vi "write_text_file_temp.vi"(0 "counts":i32=124928 caption="photon count", 1 "name":string, 2 "base path":path) -> ()   [LabVIEW 2013]
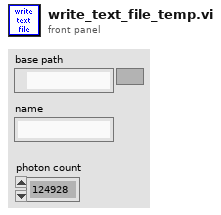
[diagram p1: front panel]
types:
  T1 = enum16{"open", "replace", "create", "open or create", "replace or create", "replace or create with confirmation"}
  T2 = cluster{"Xpixels":i32, "Vx-min ref":dbl, "Vx-max ref":dbl, "P":dbl, "Ypixels":i32, "Vy-min ref":dbl, "Vy-max ref":dbl, "srate":sgl, "sAOxy":i32, "timeout":dbl, "type":string, "date":string, "time":string, "Colormap":u16, "Drawing Mode":u16, "Scanning Mode":u16, "square pixels":bool, "square matrix":bool, "Xpixels Img":i32, "Vx-min Img":dbl, "VX-max Img":dbl, "Ypixels Img":i32, "Vy-min Img":dbl, "Vy-max Img ":dbl, "Angle Img":dbl, "autoshutter":bool, "finite":bool, "cont":bool, "wavdet":bool, "measpoints":i32, "avpp":i32, "bufferAO":i32, "bufferAI":i32, "CH1":bool, "CH2":bool, "X":bool, "Y":bool, "Ip":bool, "Vp":bool, "starttick":u32, "waveform":path, "Vx-ref":dbl, "Vy-ref":dbl, "refreshrate":dbl, "refreshbuffer":i32, "tt_cycles":i32, "motorref":refnum<k7>, "mirrorswitch":refnum<k7>, "sample mode":i32, "maxbufferAI":i32, "sampletreshold":dbl}
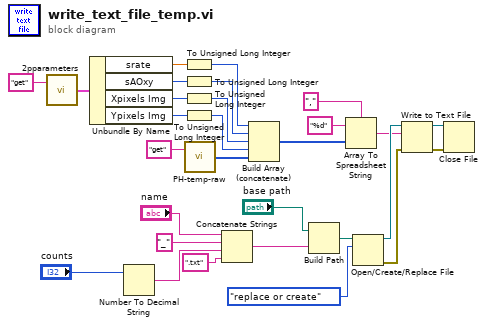
[diagram p0: block diagram]
diagram:
  n1 = call "2pparameters.vi"("command"="get") -> ("Params out"=w12:T2)  [unwired: 1 in]
  n2 = Unbundle By Name(w12) -> ("srate"=w8:sgl, "sAOxy"=w7:i32, "Xpixels Img"=w5:i32, "Ypixels Img"=w3:i32)
  n3 = Number To Decimal String(number="counts") -> (decimal integer string=w15:string)  [unwired: 1 in]
  n4 = To Unsigned Long Integer(number=w8) -> (unsigned 32bit integer=w10:u32)
  n5 = To Unsigned Long Integer(number=w7) -> (unsigned 32bit integer=w6:u32)
  n6 = To Unsigned Long Integer(number=w5) -> (unsigned 32bit integer=w4:u32)
  n7 = To Unsigned Long Integer(number=w3) -> (unsigned 32bit integer=w2:u32)
  n8 = call "PH-temp-raw.vi"("command"="get") -> ("array out"=w1:u32[])  [unwired: 1 in]
  n9 = Concatenate Strings("name", "_" ("command"), w15, ".txt" ("string")) -> (w20:string)
  n10 = Build Array (concatenate)(w10, w6, w4, w2, w1) -> (w11:u32[])
  n11 = Build Path(base path="base path", name or relative path=w20) -> (appended path=w18:path)
  n12 = Array To Spreadsheet String(delimiter (Tab)=",", array=w11, 3:"%d" ("format string")) -> (spreadsheet string=w21:string)
  n13 = Open/Create/Replace File(file path (use dialog)=w18, operation (0:open)=T1."replace or create") -> (refnum out=w29:refnum<file>, error out=w26:errorcluster)  [unwired: 4 in, 1 out]
  n14 = Write to Text File(file (use dialog)=w29, text=w21, error in=w26) -> (refnum out=w28:refnum<file>, error out=w27:errorcluster)  [unwired: 1 in, 1 out]
  n15 = Close File(refnum=w28, error in=w27) -> ()  [unwired: 2 out]
